vi "Add State to Routing Channel.vi"(8 "error in (no error)":errorcluster, 9 "Value":dbl, 10 "State":string, 11 "Channel Ref in":T1 format="%.0x") -> (0 "error out":errorcluster, 3 "Channel Ref out":T1=18446744073709551615 format="%.0x")   [LabVIEW 2017, in "Switch Scripting.lvlib"]
uses:
  Switch Scripting.lvlib
  <vilib>/NI Veristand/Custom Device API/Custom Device Item Ref.ctl
  <vilib>/NI VeriStand/Custom Device API/Custom Device API.lvlib
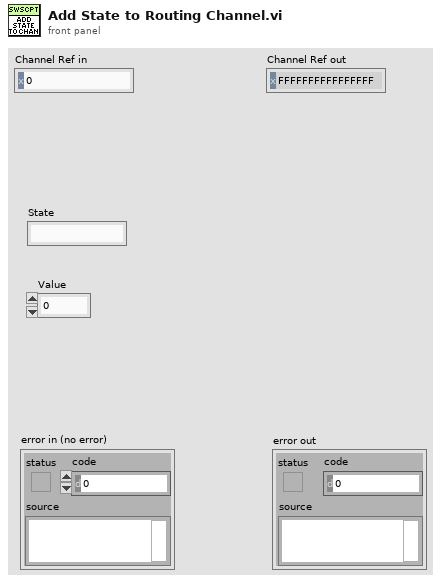
[diagram p1: front panel]
types:
  T1 = typedef "Custom Device API.lvlib/Custom Device Item Ref.ctl" = u64
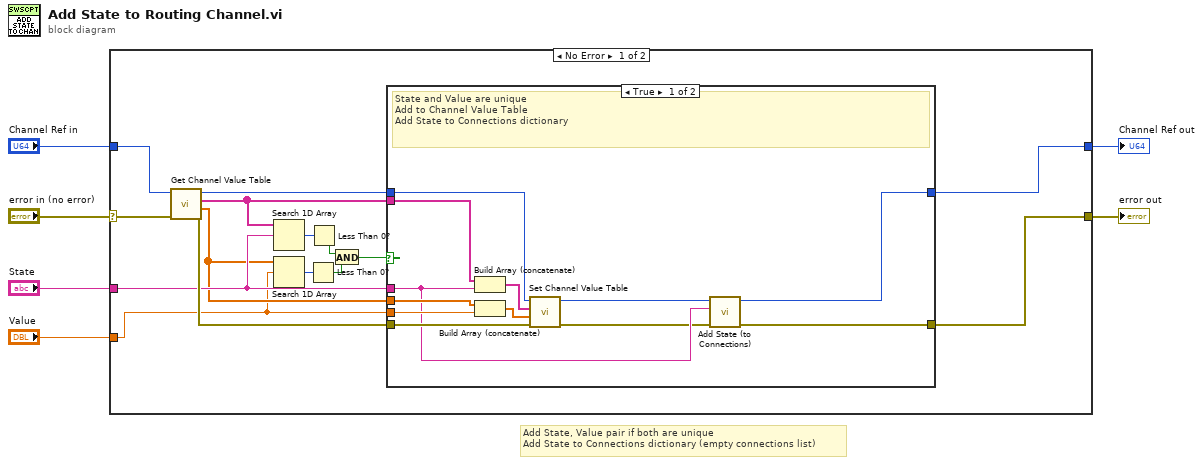
[diagram p0: block diagram]
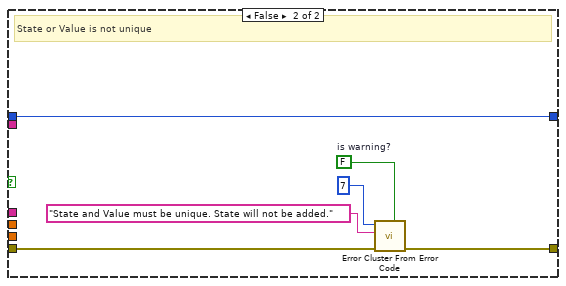
[diagram p2: hidden frame]
diagram:
  # "Add State, Value pair if both are unique\nAdd State to Connections dictionary (empty connections list)"
  n1 = case shown="No Error" "error in (no error)" {
    selector: "error in (no error)" -> [w20 w41]
    tunnel: [w16 w41] -> w2
    tunnel: "Channel Ref in" -> [w21 w40]
    tunnel: [w17 w40] -> w4
    tunnel: "State" -> [w14 _]
    tunnel: "Value" -> [w12 _]
    frame No Error {
      n2 = call "Get Channel Value Table.vi"("error in (no error)"=w20, "Channel Ref in"=w21) -> ("error out"=w18:errorcluster, "Values"=w13:dbl[], "States"=w15:string[], "Channel Ref out"=w19:T1)  [unwired: 6 in]
      n3 = Search 1D Array(1D array=w15, element=w14) -> (index of element=w11:i32)  [unwired: 1 in]
      n4 = Search 1D Array(1D array=w13, element=w12) -> (index of element=w10:i32)  [unwired: 1 in]
      n5 = Less Than 0?(x=w10) -> (x < 0?=w8:bool)
      n6 = Less Than 0?(x=w11) -> (x < 0?=w9:bool)
      n7 = And(x=w9, y=w8) -> (x .and. y?=w7:bool)
      n8 = case shown="True" w7 {
        tunnel: w19 -> [w30 w34]
        tunnel: w18 -> [w29 w36]
        tunnel: w13 -> [w32 _]
        tunnel: [w25 w34] -> w17
        tunnel: [w22 w35] -> w16
        tunnel: w12 -> [w33 _]
        tunnel: w15 -> [w31 _]
        tunnel: w14 -> [w24 _]
        frame True {
          # "State and Value are unique\nAdd to Channel Value Table\nAdd State to Connections dictionary"
          n9 = Build Array (concatenate)(w31, w24) -> (w28:string[])
          n10 = Build Array (concatenate)(w32, w33) -> (w27:dbl[])
          n11 = call "Set Channel Value Table.vi"("error in (no error)"=w29, "Values"=w27, "States"=w28, "Channel Ref in"=w30) -> ("error out"=w23:errorcluster, "Channel Ref out"=w26:T1)  [unwired: 6 in]
          n12 = call "Add State (to Connections).vi"("error in (no error)"=w23, "State"=w24, "Channel Ref in"=w26) -> ("error out"=w22:errorcluster, "Channel Ref out"=w25:T1)  [unwired: 7 in]
        }
        frame False {
          w38 = FALSE  # is warning?
          # "State or Value is not unique"
          n13 = call <vilib>:"Error Cluster From Error Code.vi"("is warning? (False)"=w38, "error in (no error)"=w36, "error message (\"\")"="State and Value must be unique. State will not be added." ("error message (\"\")"), "error code (0)"=7) -> ("error out"=w35:errorcluster)  [unwired: 5 in]
        }
      }
    }
    frame Error {
    }
  }
  "Channel Ref out" <- w4
  "error out" <- w2
